vi "AlAs_GaAs_wait_SL2.vi"(2 "Debug Mode":bool, 3 "Elapsed Time(s)":dbl, 4 "State":enum16{"Edit", "Start", "Run", "End", "Idle"}(ring), 5 "Argument List In":string[](array[string])) -> (0 "Status Out":string, 1 "Argument List Out":string[](array[string]))   [LabVIEW 2011]
panel:
  in  "tAl wait (s)":dbl
  in  "tAl flow (s)":dbl
  in  "Al flow (sccm)":dbl
  in  "nPeriods":dbl
  out "tTotal(s)":dbl
  out "tPeriod(s)":dbl
  in  "tGa wait (s)":dbl
  in  "tGa flow (s)":dbl
  in  "Ga flow (sccm)":dbl
  in  "Cancel":bool
  in  "OK":bool
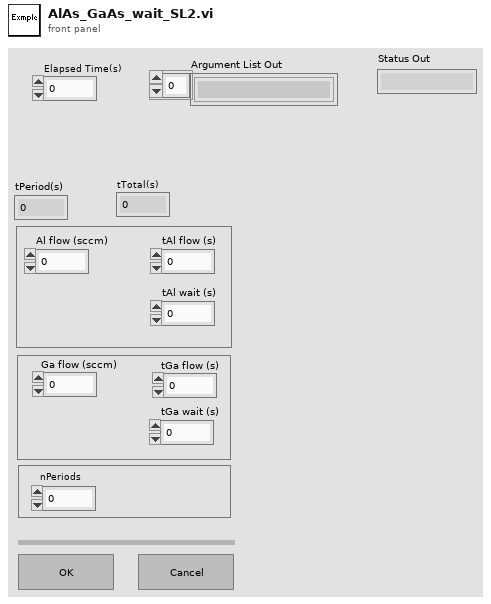
[diagram p1: front panel]
types:
  T1 = enum16{"Discrete", "Continuous", "Instantaneous"}
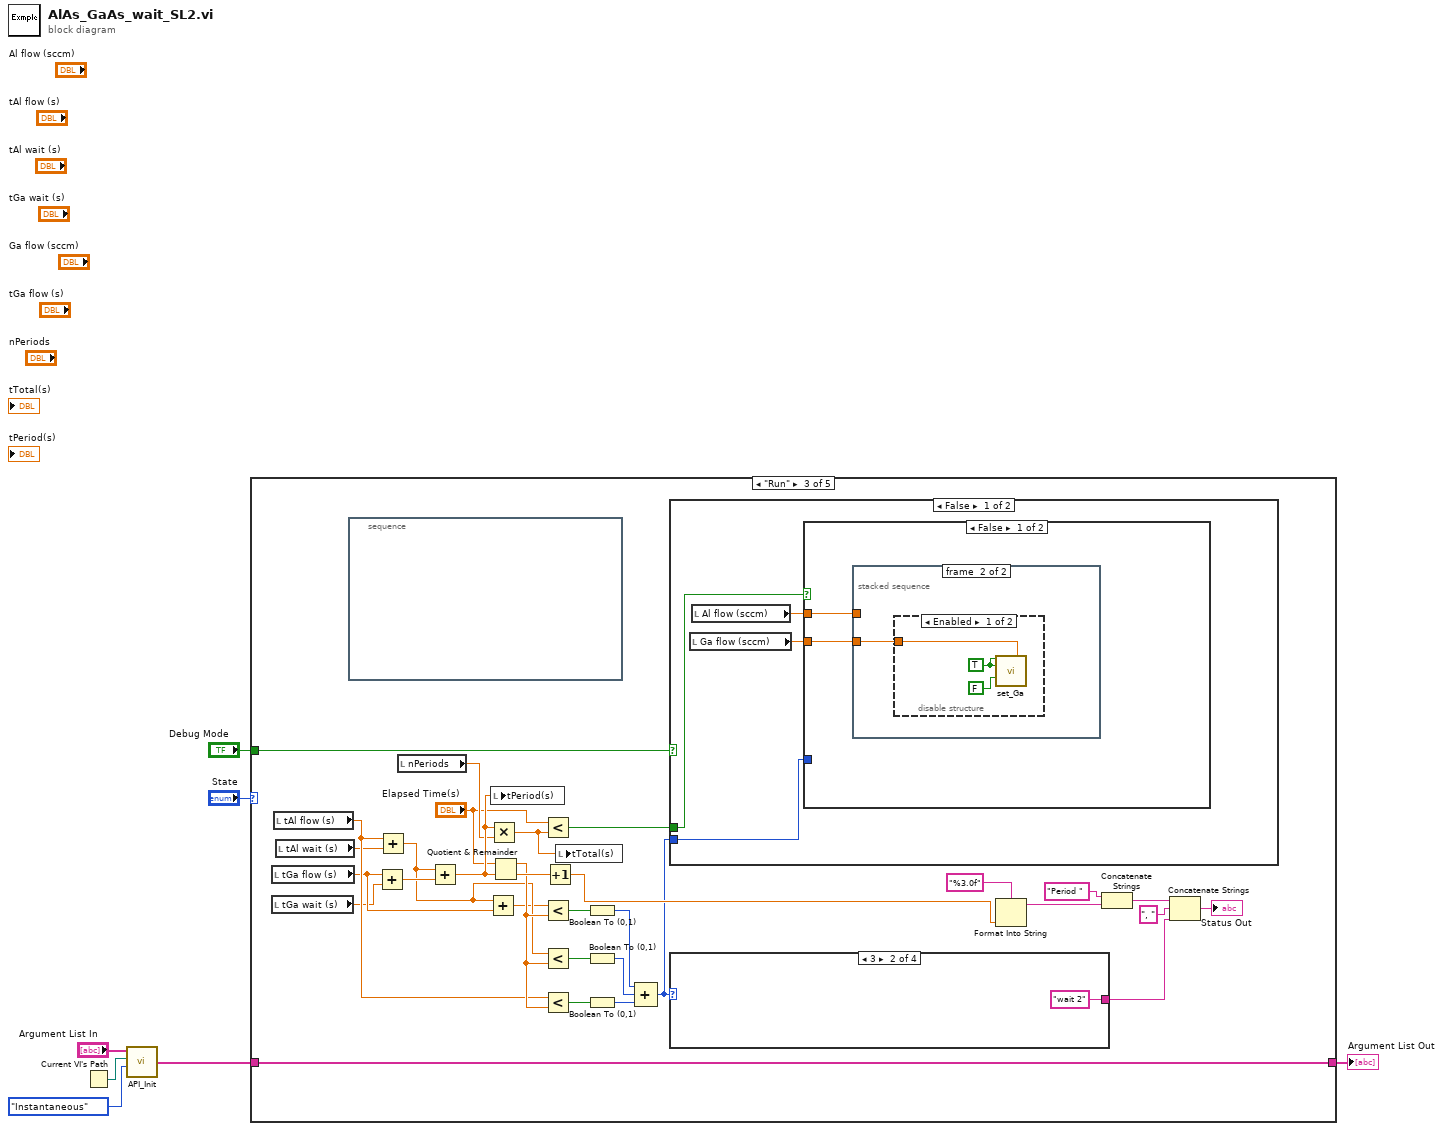
[diagram p0: block diagram]
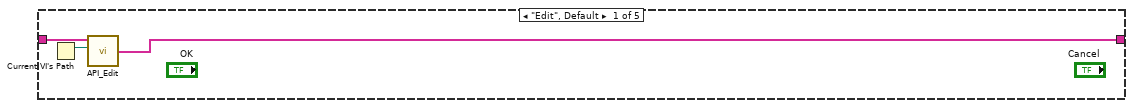
[diagram p2: hidden frame]
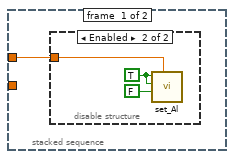
[diagram p4: hidden frame]
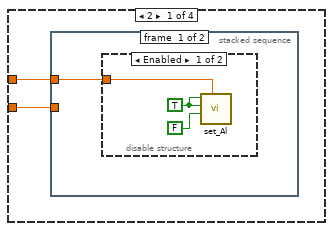
[diagram p8: hidden frame]
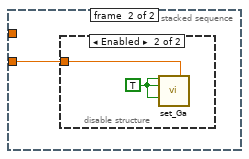
[diagram p10: hidden frame]
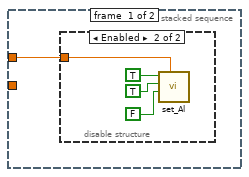
[diagram p12: hidden frame]
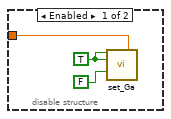
[diagram p14: hidden frame]
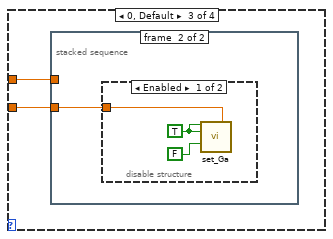
[diagram p15: hidden frame]
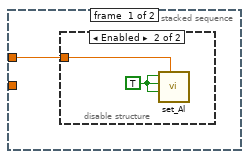
[diagram p16: hidden frame]
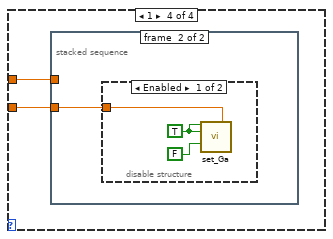
[diagram p19: hidden frame]
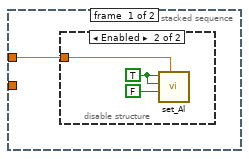
[diagram p20: hidden frame]
diagram:
  n1 = Current VI's Path() -> (path=w4:path)
  n2 = call "API_Init.vi"("API Mode"=T1."Instantaneous", "VI Path"=w4, "Argument List In"="Argument List In") -> ("Argument List Out"=w5:string[])  [unwired: 1 in]
  n3 = case shown="\"Run\"" "State" {
    tunnel: [w8 w11 w17 w113 w114] -> w1
    tunnel: w5 -> [w10 w11 w17 w113 w114]
    tunnel: "Debug Mode" -> [_ _ w18 _ _]
    frame "Edit", Default {
      n4 = Current VI's Path() -> (path=w9:path)
      n5 = call "API_Edit.vi"("VI Path"=w9, "Argument List In"=w10) -> ("Argument List Out"=w8:string[])  [unwired: 2 in]
    }
    frame "Start" {
    }
    frame "Run" {
      n6 = local read "tGa flow (s)"() -> (w20:dbl)
      n7 = local read "tGa wait (s)"() -> (w19:dbl)
      n8 = local read "tAl flow (s)"() -> (w22:dbl)
      n9 = local read "tAl wait (s)"() -> (w21:dbl)
      n10 = stacked-sequence {
        frame #0 {
        }
      }
      n11 = Add(x=w20, y=w19) -> (x+y=w35:dbl)
      n12 = Add(x=w22, y=w21) -> (x+y=w33:dbl)
      n13 = local read "nPeriods"() -> (w15:dbl)
      n14 = Add(x=w33, y=w35) -> (x+y=w16:dbl)
      n15 = Add(x=w33, y=w20) -> (x+y=w32:dbl)
      n16 = Multiply(x=w16, y=w15) -> (x*y=w13:dbl)
      n17 = local write "tPeriod(s)"(w16) -> ()
      n18 = Quotient & Remainder(x="Elapsed Time(s)", y=w16) -> (x-y*floor(x/y)=w34:dbl, floor(x/y)=w36:dbl)
      n19 = Less?(x="Elapsed Time(s)", y=w13) -> (x < y?=w12:bool)
      n20 = Less?(x=w32, y=w34) -> (x < y?=w27:bool)
      n21 = Less?(x=w33, y=w34) -> (x < y?=w29:bool)
      n22 = Less?(x=w22, y=w34) -> (x < y?=w31:bool)
      n23 = Increment(x=w36) -> (x+1=w39:dbl)
      n24 = local write "tTotal(s)"(w13) -> ()
      n25 = Boolean To (0,1)(Boolean=w27) -> (0, 1=w26:i16)
      n26 = Boolean To (0,1)(Boolean=w29) -> (0, 1=w28:i16)
      n27 = Boolean To (0,1)(Boolean=w31) -> (0, 1=w30:i16)
      n28 = Compound Arithmetic op=ADD(w26, w28, w30) -> (w24:i16)
      n29 = case shown="False" w18 {
        tunnel: w24 -> [w46 _]
        tunnel: w12 -> [w45 _]
        frame False {
          n30 = local read "Ga flow (sccm)"() -> (w44:dbl)
          n31 = local read "Al flow (sccm)"() -> (w43:dbl)
          n32 = case shown="False" w45 {
            tunnel: w46 -> [_ w59]
            tunnel: w44 -> [w47 w58]
            tunnel: w43 -> [w48 w57]
            frame False {
              n33 = stacked-sequence {
                tunnel: w48 -> [w49 _]
                tunnel: w47 -> [_ w53]
                frame #0 {
                  n34 = disable-structure shown="Enabled" {
                    disable-tunnel: w49 -> [_ w52]
                    frame Disabled {
                    }
                    frame Enabled {
                      w51 = TRUE ("Al Active")
                      n35 = call "set_Al.vi"("Aluminum Flow"=w52, "Al Run"=FALSE, "Al Bubbler"=w51, "Al Active"=w51) -> ()  [unwired: 6 in]
                    }
                  }
                }
                frame #1 {
                  n36 = disable-structure shown="Enabled" {
                    disable-tunnel: w53 -> [w54 _]
                    frame Enabled {
                      w55 = TRUE ("Ga Active")
                      n37 = call "set_Ga.vi"("Ga Active"=w55, "Ga Flow 1"=w54, "Ga Bubbler"=w55, "Ga Run"=FALSE) -> ()  [unwired: 4 in, 8 out]
                    }
                    frame Disabled {
                    }
                  }
                }
              }
            }
            frame True {
              n38 = case shown="3" w59 {
                tunnel: w57 -> [w61 w70 w81 w90]
                tunnel: w58 -> [w60 w69 w80 w89]
                frame 2 {
                  n39 = stacked-sequence {
                    tunnel: w61 -> [w62 _]
                    tunnel: w60 -> [_ w66]
                    frame #0 {
                      n40 = disable-structure shown="Enabled" {
                        disable-tunnel: w62 -> [w63 _]
                        frame Enabled {
                          w65 = TRUE ("Ga Active")
                          n41 = call "set_Al.vi"("Aluminum Flow"=w63, "Al Run"=FALSE, "Al Bubbler"=w65, "Al Active"=w65) -> ()  [unwired: 6 in]
                        }
                        frame Disabled {
                        }
                      }
                    }
                    frame #1 {
                      n42 = disable-structure shown="Enabled" {
                        disable-tunnel: w66 -> [_ w68]
                        frame Disabled {
                        }
                        frame Enabled {
                          w67 = TRUE ("Ga Active")
                          n43 = call "set_Ga.vi"("Ga Active"=w67, "Ga Flow 1"=w68, "Ga Bubbler"=w67, "Ga Run"=w67) -> ()  [unwired: 12 in]
                        }
                      }
                    }
                  }
                }
                frame 3 {
                  n44 = stacked-sequence {
                    tunnel: w70 -> [w71 _]
                    tunnel: w69 -> [_ w76]
                    frame #0 {
                      n45 = disable-structure shown="Enabled" {
                        disable-tunnel: w71 -> [_ w72]
                        frame Disabled {
                        }
                        frame Enabled {
                          n46 = call "set_Al.vi"("Aluminum Flow"=w72, "Al Run"=FALSE, "Al Bubbler"=TRUE, "Al Active"=TRUE) -> ()  [unwired: 6 in]
                        }
                      }
                    }
                    frame #1 {
                      n47 = disable-structure shown="Disabled" {
                        disable-tunnel: w76 -> [w77 _]
                        frame Enabled {
                          w78 = TRUE ("Ga Active")
                          n48 = call "set_Ga.vi"("Ga Active"=w78, "Ga Flow 1"=w77, "Ga Bubbler"=w78, "Ga Run"=FALSE) -> ()  [unwired: 4 in, 8 out]
                        }
                        frame Disabled {
                        }
                      }
                    }
                  }
                }
                frame 0, Default {
                  n49 = stacked-sequence {
                    tunnel: w81 -> [w82 _]
                    tunnel: w80 -> [_ w85]
                    frame #0 {
                      n50 = disable-structure shown="Enabled" {
                        disable-tunnel: w82 -> [_ w84]
                        frame Disabled {
                        }
                        frame Enabled {
                          w83 = TRUE ("Al Active")
                          n51 = call "set_Al.vi"("Aluminum Flow"=w84, "Al Run"=w83, "Al Bubbler"=w83, "Al Active"=w83) -> ()  [unwired: 6 in]
                        }
                      }
                    }
                    frame #1 {
                      n52 = disable-structure shown="Enabled" {
                        disable-tunnel: w85 -> [w86 _]
                        frame Enabled {
                          w87 = TRUE ("Ga Active")
                          n53 = call "set_Ga.vi"("Ga Active"=w87, "Ga Flow 1"=w86, "Ga Bubbler"=w87, "Ga Run"=FALSE) -> ()  [unwired: 4 in, 8 out]
                        }
                        frame Disabled {
                        }
                      }
                    }
                  }
                }
                frame 1 {
                  n54 = stacked-sequence {
                    tunnel: w89 -> [_ w95]
                    tunnel: w90 -> [w91 _]
                    frame #0 {
                      n55 = disable-structure shown="Enabled" {
                        disable-tunnel: w91 -> [_ w93]
                        frame Disabled {
                        }
                        frame Enabled {
                          w92 = TRUE ("Al Bubbler")
                          n56 = call "set_Al.vi"("Aluminum Flow"=w93, "Al Run"=FALSE, "Al Bubbler"=w92, "Al Active"=w92) -> ()  [unwired: 6 in]
                        }
                      }
                    }
                    frame #1 {
                      n57 = disable-structure shown="Enabled" {
                        disable-tunnel: w95 -> [w96 _]
                        frame Enabled {
                          w97 = TRUE ("Ga Active")
                          n58 = call "set_Ga.vi"("Ga Active"=w97, "Ga Flow 1"=w96, "Ga Bubbler"=w97, "Ga Run"=FALSE) -> ()  [unwired: 4 in, 8 out]
                        }
                        frame Disabled {
                        }
                      }
                    }
                  }
                }
              }
            }
          }
        }
        frame True {
        }
      }
      n59 = case shown="3" w24 {
        tunnel: [w100 "wait 2" w107 "wait 1"] -> w25
        frame 2 {
          n60 = local read "Ga flow (sccm)"() -> (w99:dbl)
          n61 = Format Into String(format string="%4.2f", w99) -> (resulting string=w103:string)  [unwired: 2 in, 1 out]
          n62 = Concatenate Strings("Ga(" ("string"), w103, "sccm)" ("string")) -> (w100:string)
        }
        frame 3 {
        }
        frame 0, Default {
          n63 = local read "Al flow (sccm)"() -> (w106:dbl)
          n64 = Format Into String(format string="%4.1f", w106) -> (resulting string=w109:string)  [unwired: 2 in, 1 out]
          n65 = Concatenate Strings("Al(" ("string"), w109, "sccm)" ("string")) -> (w107:string)
        }
        frame 1 {
        }
      }
      n66 = Format Into String(format string="%3.0f", w39) -> (resulting string=w40:string)  [unwired: 2 in, 1 out]
      n67 = Concatenate Strings("Period " ("string"), w40) -> (w37:string)
      n68 = Concatenate Strings(w37, ", " ("string"), w25) -> (→"Status Out":string)
    }
    frame "End" {
    }
    frame "Idle" {
    }
  }
  "Argument List Out" <- w1
